vi "Lesson3 - Explicit Property Node SubVI.vi"(9 "Vertical Fill Slide in":dbl, 10 "Bool Refnum":refnum<vi>, 11 "Slide in":refnum<vi>) -> ()   [LabVIEW 2013]
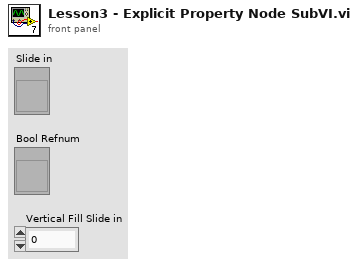
[diagram p1: front panel]
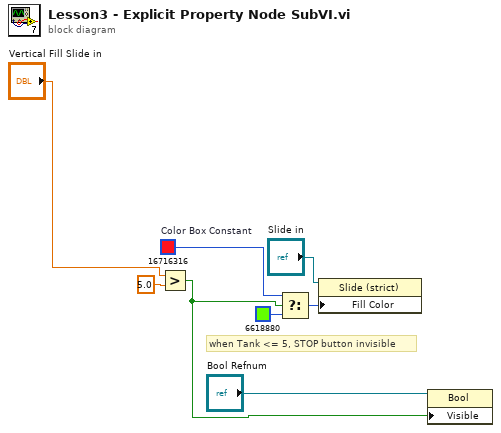
[diagram p0: block diagram]
diagram:
  w5 = u32 16716316  # Color Box Constant
  # "when Tank <= 5, STOP button invisible"
  n1 = Greater?(x="Vertical Fill Slide in", y=5.0) -> (0:w8:bool)
  n2 = Select(t=w5, s=w8, f=u32 6618880) -> (s? t:f=w7:u32)
  n3 = property on="Property Node" class="Slide (strict)"(reference="Slide in", "Fill Color"=w7) -> ()  [unwired: 1 in, 2 out]
  n4 = property on="Property Node" class="Bool"(reference="Bool Refnum", "Visible"=w8) -> ()  [unwired: 1 in, 2 out]
